vi "CRYUpdate Operator Close All Menu.vi"   [LabVIEW 2013]
uses:
  SubVI/CRYMain Sub Window Global.vi
  CRYSystem/Misc/SubVI/CRYMisc vis settings global.vi
types:
  T1 = cluster{"VI Ref":refnum<vi>[], "VI nID":i32[], "Title nID":i32[]}
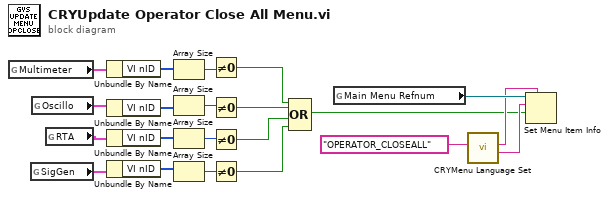
[diagram p0: block diagram]
diagram:
  n1 = global read "CRYMisc vis settings global.vi" "Multimeter"() -> (w21:T1)
  n2 = global read "CRYMisc vis settings global.vi" "SigGen"() -> (w17:T1)
  n3 = global read "CRYMisc vis settings global.vi" "Oscillo"() -> (w19:T1)
  n4 = global read "CRYMisc vis settings global.vi" "RTA"() -> (w18:T1)
  n5 = Unbundle By Name(w21) -> ("VI nID"=w20:i32[])
  n6 = Unbundle By Name(w19) -> ("VI nID"=w16:i32[])
  n7 = Unbundle By Name(w18) -> ("VI nID"=w15:i32[])
  n8 = Unbundle By Name(w17) -> ("VI nID"=w14:i32[])
  n9 = Array Size(array=w20) -> (size(s)=w13:i32)
  n10 = Array Size(array=w16) -> (size(s)=w12:i32)
  n11 = Array Size(array=w15) -> (size(s)=w11:i32)
  n12 = Array Size(array=w14) -> (size(s)=w10:i32)
  n13 = Not Equal To 0?(x=w13) -> (x != 0?=w9:bool)
  n14 = Not Equal To 0?(x=w12) -> (x != 0?=w8:bool)
  n15 = Not Equal To 0?(x=w11) -> (x != 0?=w7:bool)
  n16 = Not Equal To 0?(x=w10) -> (x != 0?=w6:bool)
  n17 = Compound Arithmetic op=OR(w9, w8, w7, w6) -> (w1:bool)
  n18 = global read "CRYMain Sub Window Global.vi" "Main Menu Refnum"() -> (w5:refnum<k9>)
  n19 = call "CRYMenu Language Set.vi"("sID"="OPERATOR_CLOSEALL" ("item tag")) -> ("sMultibyte_Out"=w2:string, "sID_Out"=w3:string)  [unwired: 7 in, 2 out]
  n20 = Set Menu Item Info(7:w3, 9:w1, 10:w2, 11:w5) -> ()  [unwired: 2 in, 3 out]
